vi "Refname to String (Actuator).vi"(1 "Actuator Refname":T1) -> (0 "Refnum Name":string)   [LabVIEW 2015]
uses:
  Refname Enum (Actuator).ctl
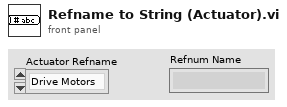
[diagram p1: front panel]
types:
  T1 = typedef "Refname Enum (Actuator).ctl" = enum16{"Drive Motors"}
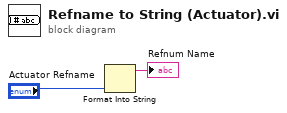
[diagram p0: block diagram]
diagram:
  n1 = Format Into String("Actuator Refname") -> (resulting string=→"Refnum Name":string)  [unwired: 3 in, 1 out]
